vi "LinearSystemLoop_New.vi"(8 "Max Input":T1, 9 "Observer":T2, 10 "FeedForward":T4, 11 "Controller":T5) -> (0 "Error":bool, 3 "Linear System Loop":T6)   [LabVIEW 2019, in "Trajectory_Library.lvlib"]
doc: "Combines a controller, feedforward, and observer for controlling a mechanism with full state feedback.\n \nFor everything in this file, \"inputs\" and \"outputs\" are defined from the perspective of the plant. This means U is an input and Y is an output (because you give the plant U (powers) and it gives you back a Y (sensor values). This is the opposite of what they mean from the perspective of the controller (U is an output because that's what goes to the motors and Y is an input because that's what comes back from the sensors).\n \nFor more on the underlying math, read https://file.tavsys.net/control/controls-engineering-in-frc.pdf.\n\nConstructs a state-space loop with the given controller, feedforward and observer. By default, the initial reference is all zeros. Users should call reset with the initial system state before enabling the loop.\n \nInputs:\n - controller -- State-space controller.\n - feedforward -- Plant inversion feedforward.\n - observer -- State-space observer.\n - maxVoltageVolts -- The maximum voltage that can be applied. Assumes that the inputs are voltages.\n\nOutputs:\n - outLinearSystemLoop -- updated system data cluster\n - error -- If TRUE, an error occured."
uses:
  Trajectory_Library.lvlib
  LINEAR_SYSTEM_LOOP.ctl
  LINEAR_QUADRATIC_REGULATOR.ctl
  <vilib>/Analysis/Matrix/Datatypes/RealMatrix.ctl
  LINEAR_PLANT_INV_FF.ctl
  KALMAN_FILTER.ctl
  LINEAR_SYSTEM.ctl
  <vilib>/Analysis/Matrix/NI_Matrix.lvlib
panel:
  # "Steady State Gain  \n<States,Outputs>"
  # "State Estimate <Statess,1>"
  # "<States,States>"
  # "<States,Inputs>"
  # "<Outputs,States>"
  # "<Outputs,Inputs>"
  # "<States,1>"
  # "<Inputs,1>"
  # "<States,Inputs>"
  # "<States,States>"
  # "Ref State <States,1>"
  # "Comp and capped \noutput <Inputs,1>"
  # "Controller gain\n<Inputs,States>"
  # "<States,1>"
  # "<FUTURE --- CLAMP TYPE -- For now\nuse Normalize>"
  # "Steady State Gain  \n<States,Outputs>"
  # "State Estimate <Statess,1>"
  # "<States,States>"
  # "<States,Inputs>"
  # "<Outputs,States>"
  # "<Outputs,Inputs>"
  # "<States,1>"
  # "<Inputs,1>"
  # "<States,Inputs>"
  # "<States,States>"
  # "Ref State <States,1>"
  # "Comp and capped \noutput <Inputs,1>"
  # "Controller gain\n<Inputs,States>"
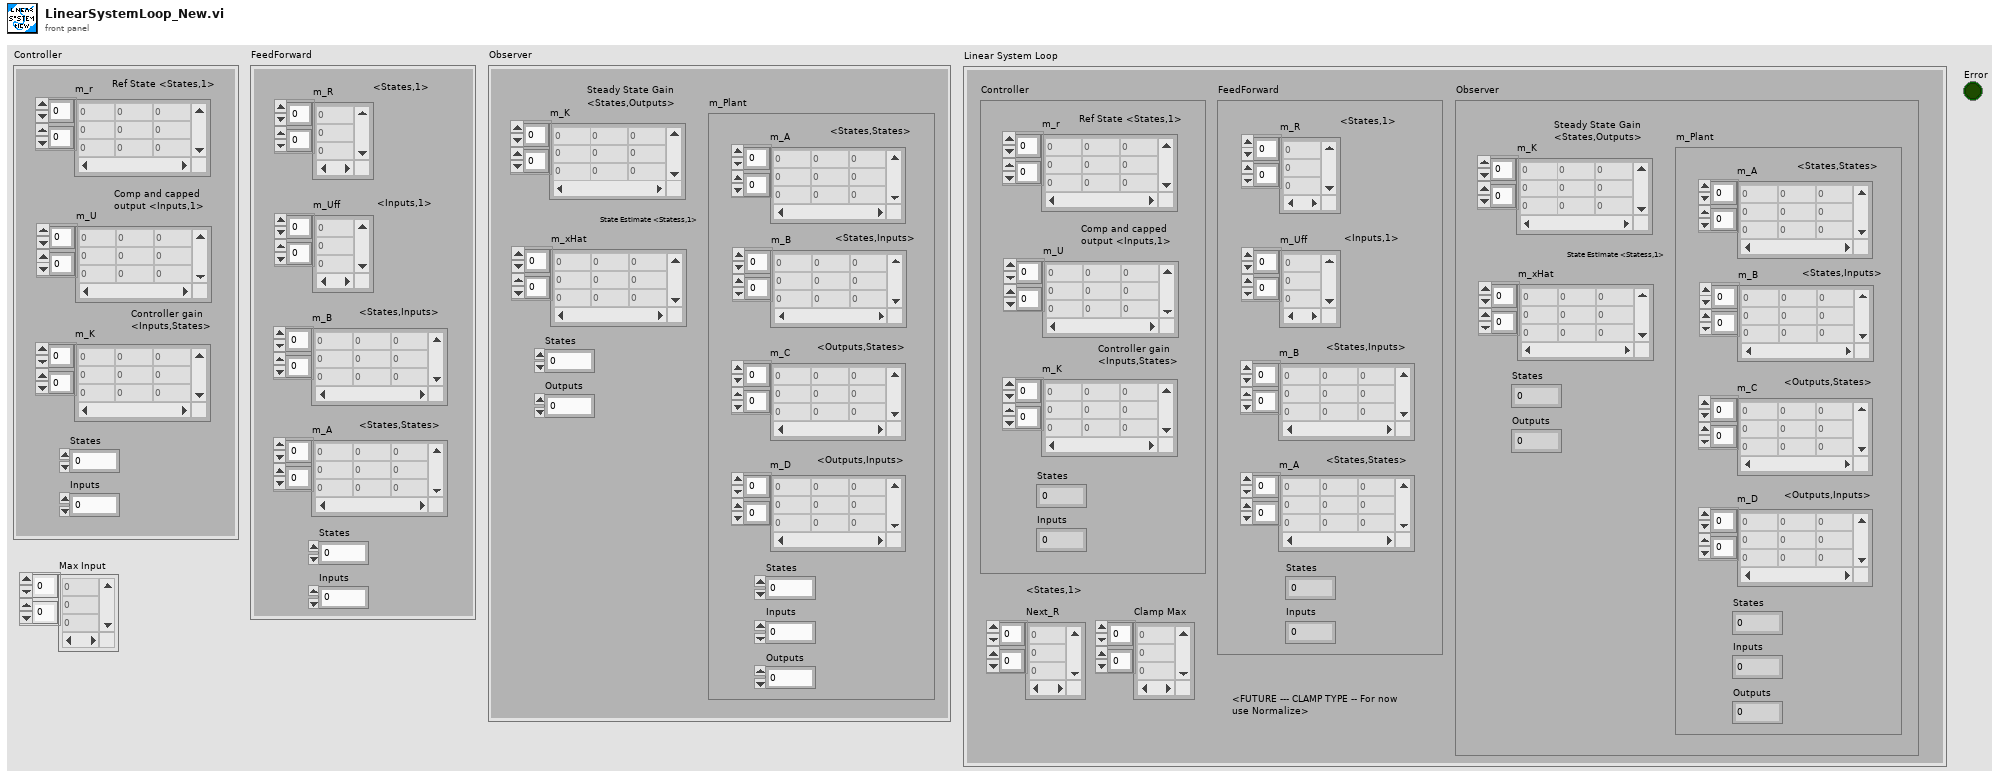
[diagram p1: front panel]
types:
  T1 = typedef "NI_Matrix.lvlib/RealMatrix.ctl" = dbl[][]
  T2 = typedef "Trajectory_Library.lvlib/KALMAN_FILTER.ctl" = cluster{"m_K":T1, "m_xHat":T1, "States":i32, "Outputs":i32, "m_Plant":T3}
  T3 = typedef "Trajectory_Library.lvlib/LINEAR_SYSTEM.ctl" = cluster{"m_A":T1, "m_B":T1, "m_C":T1, "m_D":T1, "States":i32, "Inputs":i32, "Outputs":i32}
  T4 = typedef "Trajectory_Library.lvlib/LINEAR_PLANT_INV_FF.ctl" = cluster{"m_R":T1, "m_Uff":T1, "m_B":T1, "m_A":T1, "States":i32, "Inputs":i32}
  T5 = typedef "Trajectory_Library.lvlib/LINEAR_QUADRATIC_REGULATOR.ctl" = cluster{"m_r":T1, "m_U":T1, "m_K":T1, "States":i32, "Inputs":i32}
  T6 = typedef "Trajectory_Library.lvlib/LINEAR_SYSTEM_LOOP.ctl" = cluster{"Controller":T5, "FeedForward":T4, "Observer":T2, "Next_R":T1, "Clamp Max":T1}
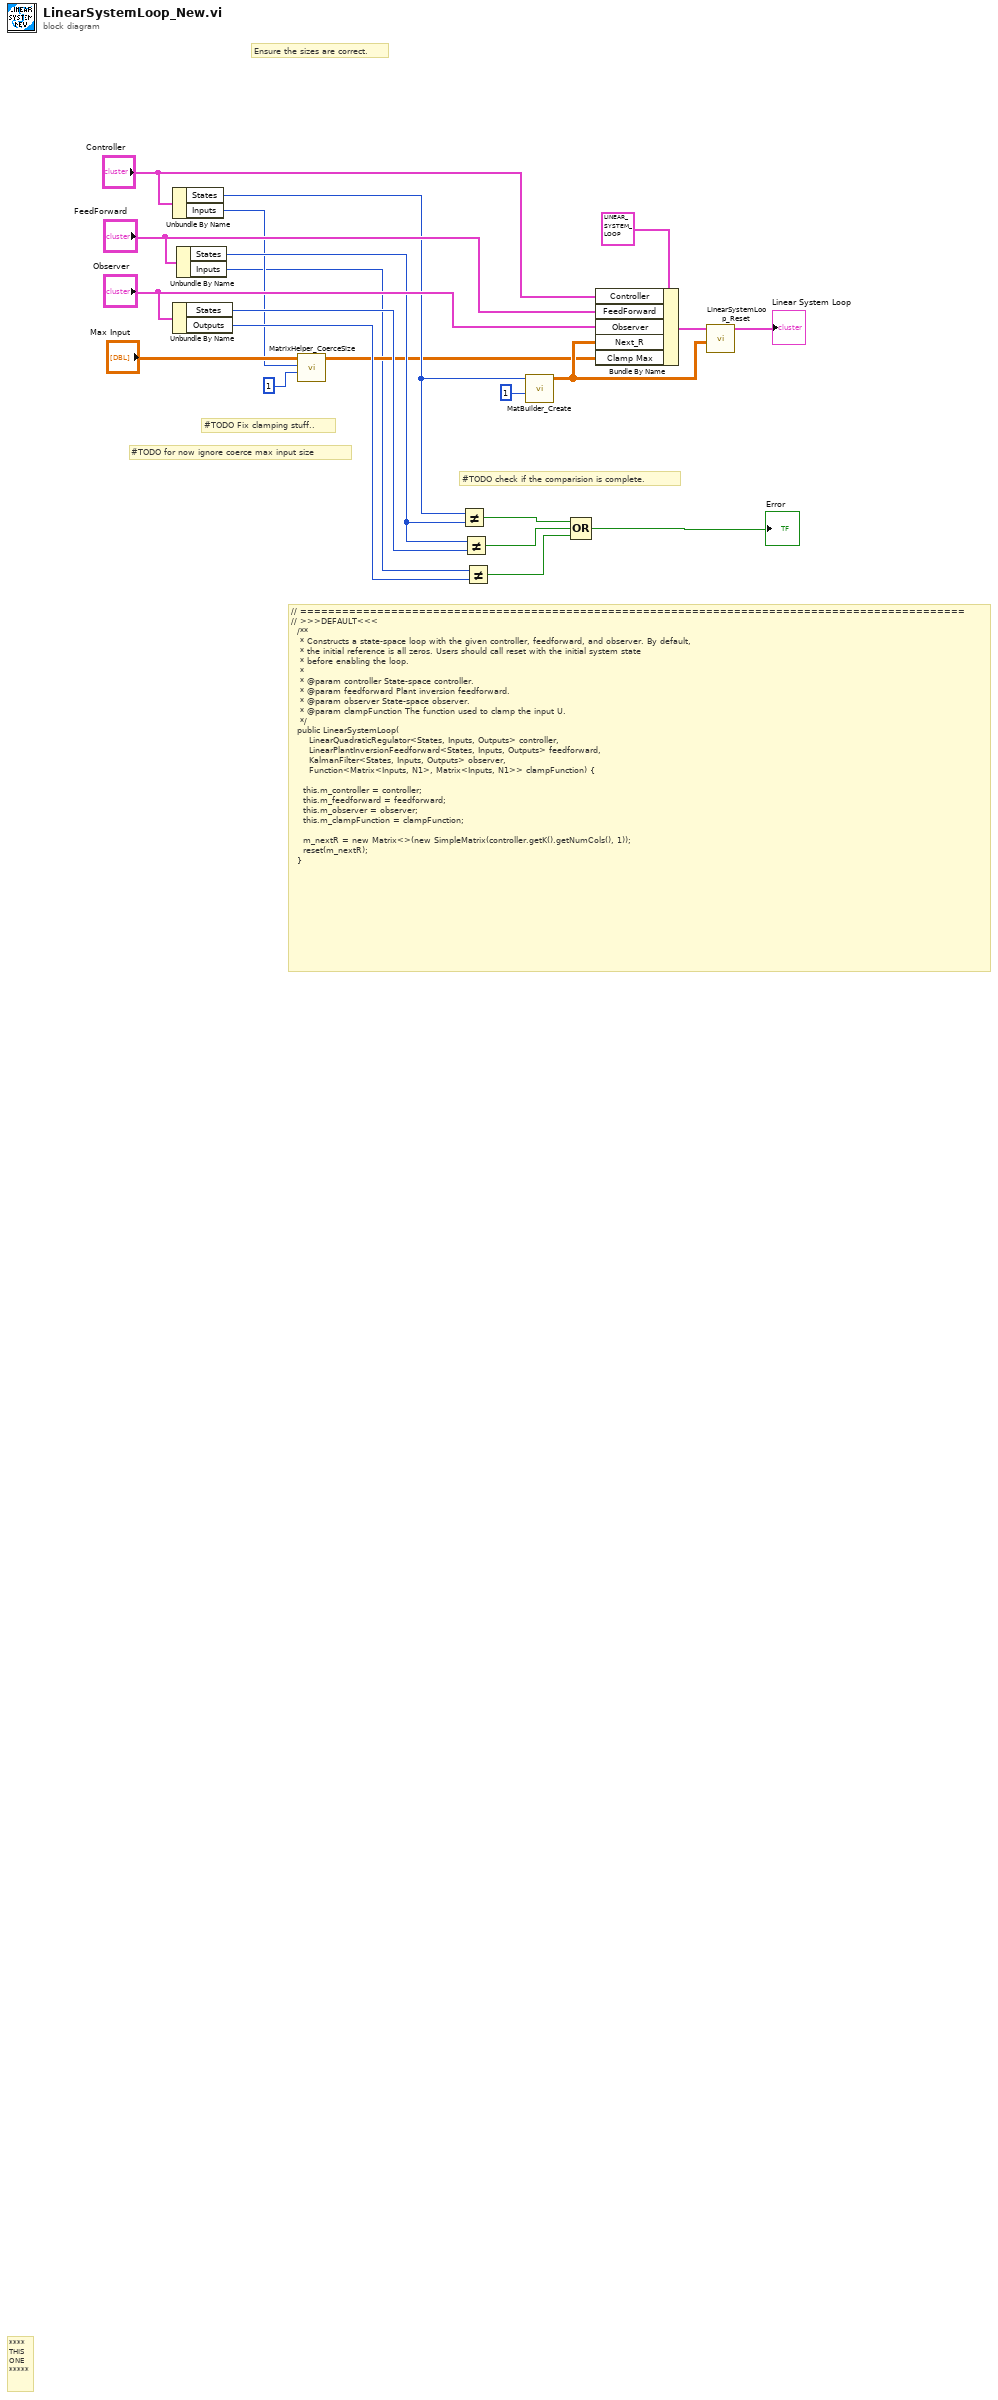
[diagram p0: block diagram]
diagram:
  # "#TODO check if the comparision is complete."
  # "#TODO for now ignore coerce max input size"
  # "#TODO Fix clamping stuff.."
  # "// ===============================================================================================\n// >>>DEFAULT<<<\n  /**\n   * Constructs a state-space loop with the given controller, feedforward, and observer. By default,\n   * the initial reference is all zeros. Users should call reset with the initial system state\n   * before enabling the loop.\n   *\n   * @param controller State-space controller.\n   * @param feedforward Plant inversion feedforward.\n   * @param observer State-space observer.\n   * @param clampFunction The function used to clamp the input U.\n   */\n  public LinearSystemLoop(\n      LinearQuadraticRegulator<States, Inputs, Outputs> controller,\n      LinearPlantInversionFeedforward<States, Inputs, Outputs> feedforward,\n      KalmanFilter<States, Inputs, Outputs> observer,\n      Function<Matrix<Inputs, N1>, Matrix<Inputs, N1>> clampFunction) {\n\n    this.m_controller = controller;\n    this.m_feedforward = feedforward;\n    this.m_observer = observer;\n    this.m_clampFunction = clampFunction;\n\n    m_nextR = new Matrix<>(new SimpleMatrix(controller.getK().getNumCols(), 1));\n    reset(m_nextR);\n  }"
  # "Ensure the sizes are correct."
  # "****\nTHIS\nONE\n*****"
  n1 = Unbundle By Name("Controller") -> ("States"=w10:i32, "Inputs"=w2:i32)
  n2 = Unbundle By Name("Observer") -> ("States"=w16:i32, "Outputs"=w15:i32)
  n3 = Unbundle By Name("FeedForward") -> ("States"=w17:i32, "Inputs"=w1:i32)
  n4 = call "MatrixHelper_CoerceSize.vi"("Columns"=1, "Rows"=w2, "input matrix"="Max Input") -> ("output matrix"=w4:T1)  [unwired: 7 in, 1 out]
  n5 = Not Equal?(x=w10, y=w17) -> (x != y?=w14:bool)
  n6 = Not Equal?(x=w17, y=w16) -> (x != y?=w13:bool)
  n7 = Not Equal?(x=w1, y=w15) -> (x != y?=w12:bool)
  n8 = call "MatBuilder_Create.vi"("Columns"=1 ("number of columns"), "Rows"=w10) -> ("output matrix"=w6:T1)  [unwired: 9 in]
  n9 = Compound Arithmetic op=OR(w14, w13, w12) -> (→"Error":bool)
  n10 = Bundle By Name(cluster=T6 {"Controller"={"m_r"=[], "m_U"=[], "m_K"=[], "States"=0, "Inputs"=0}, "FeedForward"={"m_R"=[], "m_Uff"=[], "m_B"=[], "m_A"=[], "States"=0, "Inputs"=0}, "Observer"={"m_K"=[], "m_xHat"=[], "States"=0, "Outputs"=0, "m_Plant"={"m_A"=[], "m_B"=[], "m_C"=[], "m_D"=[], "States"=0, "Inputs"=0, "Outputs"=0}}, "Next_R"=[], "Clamp Max"=[]} ("LINEAR_SYSTEM_LOOP"), "Controller"="Controller", "FeedForward"="FeedForward", "Observer"="Observer", "Next_R"=w6, "Clamp Max"=w4) -> (w8:T6)
  n11 = call "LinearSystemLoop_Reset.vi"("initialState"=w6, "input inear System Loop"=w8) -> ("out Linear System Loop"=→"Linear System Loop":T6)  [unwired: 8 in, 1 out]
